vi "Pneumatik.vi"(8 "error in (no error)":errorcluster caption="Fehler (Eingang, kein Fehler)", 9 "Single_Output":T1(ring), 10 "Module":T2(ring), 11 "Device ID":T3(ring)) -> (0 "error out":errorcluster caption="Fehler (Ausgang)", 3 "Device ID Out":T3(ring))   [LabVIEW 2010]
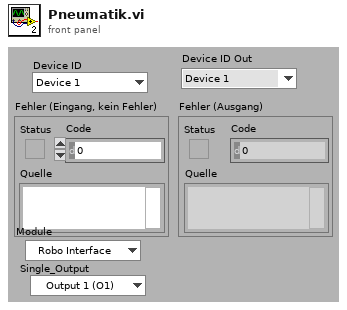
[diagram p1: front panel]
types:
  T1 = enum8{"Output 1 (O1)", "Output 2 (O2)", "Output 3 (O3)", "Output 4 (O4)", "Output 5 (O5)", "Output 6 (O6)", "Output 7 (O7)", "Output 8 (O8)"}
  T2 = enum8{"Robo Interface", "Extension 1", "Extension 2", "Extension 3"}
  T3 = enum16{"Device 1", "Device 2", "Device 3", "Device 4", "Device 5", "Device 6", "Device 7", "Device 8"}
  T4 = enum8{"Power 1", "Power 2", "Power 3", "Power 4", "Power 5", "Power 6", "Power 7", "Power 8"}
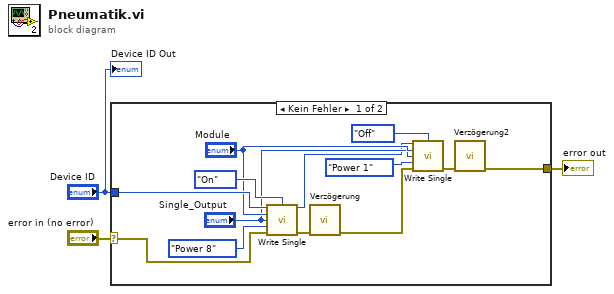
[diagram p0: block diagram]
diagram:
  n1 = case shown="Kein Fehler" "error in (no error)" {
    selector: "error in (no error)" -> [w15 w17]
    tunnel: "Device ID" -> [w16 _]
    tunnel: [w4 w17] -> w1
    frame No Error {
      n2 = call "Write Single.vi"("Device ID"=w16, "Output_Action"=enum8{"Off", "On"}."On", "Module"="Module", "Single_Output"="Single_Output", "Output_PWM"=T4."Power 8", "error in"=w15) -> ("Device ID Out"=w8:T3, "error out"=w7:errorcluster)  [unwired: 8 out]
      n3 = call "Verzögerung"("error in (no error)"=w7) -> ("error out"=w6:errorcluster)  [unwired: 1 in, 9 out]
      n4 = call "Write Single.vi"("Device ID"=w8, "Output_Action"=enum8{"Off", "On"}."Off", "Module"="Module", "Single_Output"="Single_Output", "Output_PWM"=T4."Power 1", "error in"=w6) -> ("error out"=w5:errorcluster)  [unwired: 9 out]
      n5 = call "Verzögerung2"("error in (no error)"=w5) -> ("error out"=w4:errorcluster)  [unwired: 1 in, 9 out]
    }
    frame Error {
    }
  }
  "error out" <- w1
  "Device ID Out" <- "Device ID"
